vi "Create New Tree Item.vi"(7 "Item Type":T1=enum."Group", 8 "error in":errorcluster, 9 "found?":bool, 11 "Left Cell String":string) -> (0 "error out":errorcluster, 3 "Item":T2)   [LabVIEW 2017, in "DSF Configuration Utility.lvlib"]
uses:
  DSF Configuration Utility.lvlib
  Tree Item.ctl
  ID to Tree Items/Tree Item Type.ctl
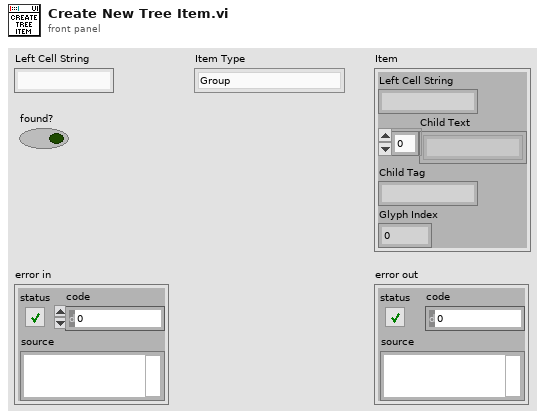
[diagram p1: front panel]
types:
  T1 = typedef "DSF Configuration Utility.lvlib/Tree Item Type.ctl" = enum16{"Plugin", "Group", "Transfer", "Channel", "Setting"}
  T2 = typedef "DSF Configuration Utility.lvlib/Tree Item.ctl" = cluster{"Left Cell String":string, "Child Text":string[], "Child Tag":string, "Glyph Index":i32}
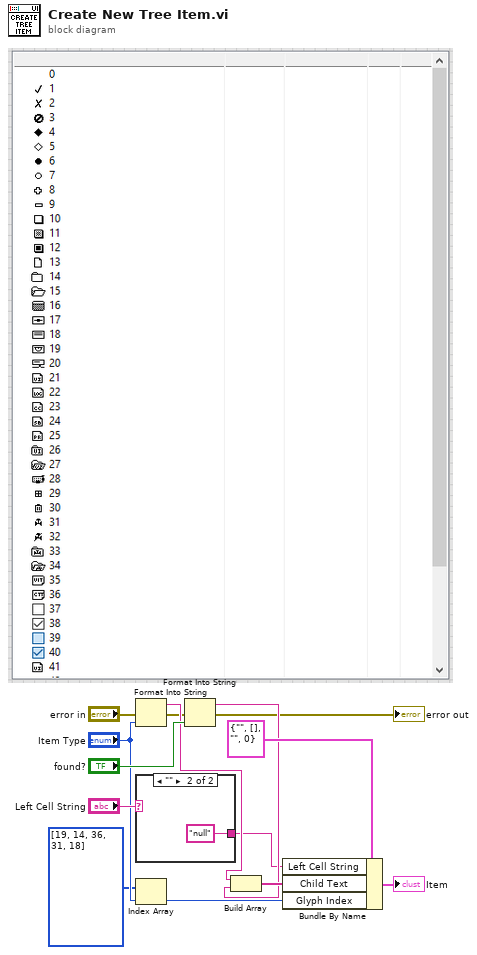
[diagram p0: block diagram]
diagram:
  n1 = Format Into String(error in="error in", "Item Type") -> (resulting string=w9:string, error out=w7:errorcluster)  [unwired: 2 in]
  n2 = case shown="\"\"" "Left Cell String" {
    selector: "Left Cell String" -> [w15 _]
    tunnel: [w15 "null"] -> w4
    frame Default {
    }
    frame "" {
    }
  }
  n3 = Index Array(array=i32[] [19, 14, 36, 31, 18] ("f"), index="Item Type") -> (element=w1:i32)
  n4 = Format Into String(error in=w7, "found?") -> (resulting string=w10:string, error out=→"error out":errorcluster)  [unwired: 2 in]
  n5 = Build Array(w9, w10) -> (w13:string[])
  n6 = Bundle By Name(cluster=T2 {"Left Cell String"="", "Child Text"=[], "Child Tag"="", "Glyph Index"=0} ("Item"), "Left Cell String"=w4, "Child Text"=w13, "Glyph Index"=w1) -> (→"Item":T2)
